vi "ATM Controller.vi"() -> ()   [LabVIEW 2012]
uses:
  DataType/ATM Controller_State.ctl
panel:
  in  "ATM Controller State":T1
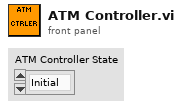
[diagram p1: front panel]
types:
  T1 = typedef "ATM Controller_State.ctl" = enum16{"Initial", "Login", "MainMenu", "Balance Inquiry", "Deposit", "Deposit Complete", "Withdrawal", "Withdrawal Success", "Withdrawal Failure", "Terminate", "Lock Out"}
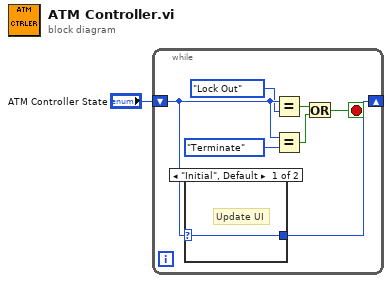
[diagram p0: block diagram]
diagram:
  n1 = while {
    shift-right: [w2] -> _
    shift-left: "ATM Controller State" -> [w7]
    stop <- w3 stop-if-true
    n2 = case shown="\"Initial\", Default" w7 {
      selector: w7 -> [w9 w10]
      tunnel: [w9 w10] -> w2
      frame "Initial", Default {
        # "Update UI"
      }
      frame "Login" {
      }
    }
    n3 = Equal?(x=w7, y=ATM_Controller_State."Lock Out") -> (x = y?=w4:bool)
    n4 = Equal?(x=w7, y=ATM_Controller_State."Terminate") -> (x = y?=w5:bool)
    n5 = Or(x=w4, y=w5) -> (x .or. y?=w3:bool)
  }
